vi "MapScriptActorGFV.vi"(8 "error in (no error)":errorcluster, 10 "MapScriptEnum":T1, 11 "Data in":variant) -> (0 "error out":errorcluster, 3 "Data Out":variant)   [LabVIEW 2017]
doc: "Use this template to build a VI to use as a subVI."
uses:
  MapScriptGFVEnum.ctl
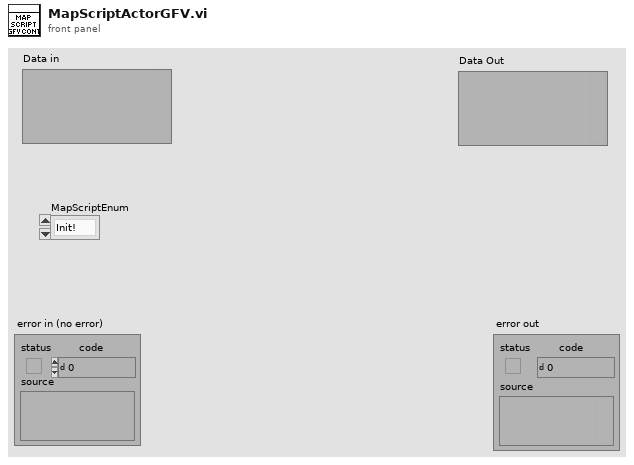
[diagram p1: front panel]
types:
  T1 = typedef "MapScriptGFVEnum.ctl" = enum16{"Init!", "Stop!", "Start!", "GetMapScriptActorViRef"}
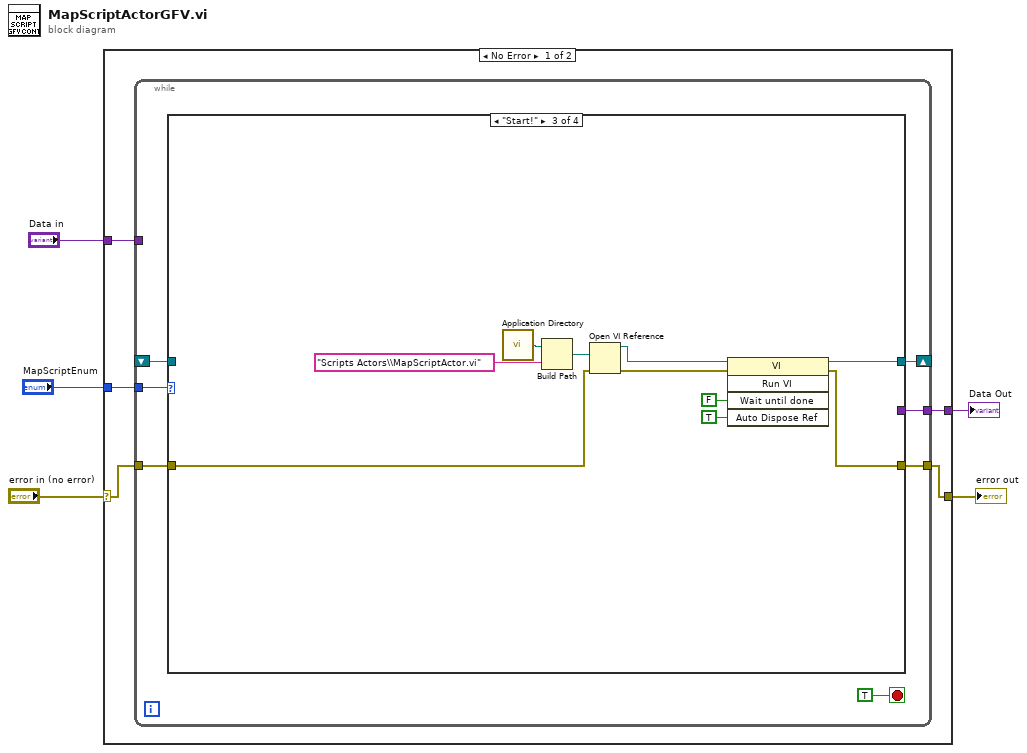
[diagram p0: block diagram]
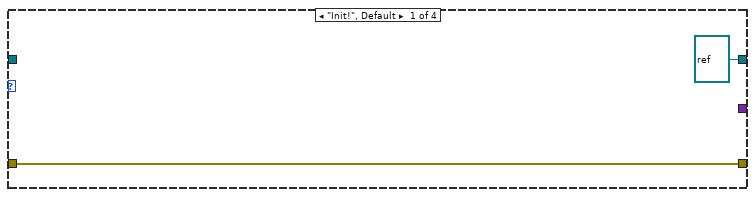
[diagram p2: hidden frame]
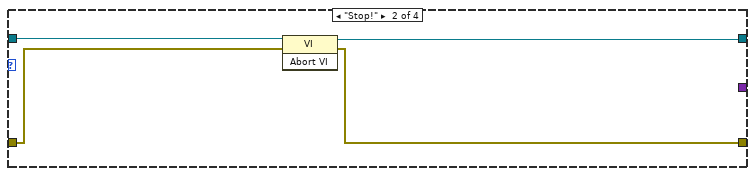
[diagram p3: hidden frame]
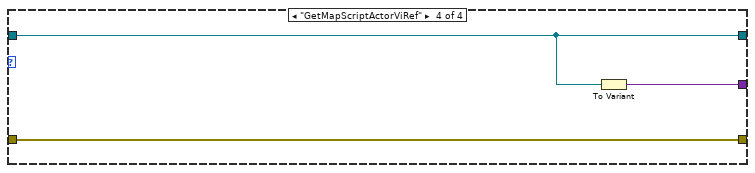
[diagram p4: hidden frame]
diagram:
  n1 = case shown="No Error" "error in (no error)" {
    selector: "error in (no error)" -> [w9 w37]
    tunnel: [w8 w37] -> w4
    tunnel: "MapScriptEnum" -> [w10 _]
    tunnel: "Data in" -> [w7 _]
    tunnel: [w6 _] -> w1
    frame No Error {
      n2 = while {
        tunnel: w10 -> [w16]
        tunnel: w9 -> [w15]
        tunnel: [w14] -> w8
        shift-right: [w13] -> _
        shift-left: _ -> [w12]
        tunnel: w7 -> [_]
        tunnel: [w11] -> w6
        stop <- TRUE stop-if-true
        n3 = case shown="\"Start!\"" w16 {
          tunnel: w15 -> [w18 w23 w26 w34]
          tunnel: [w18 w22 w25 w34] -> w14
          tunnel: [refnum<vi> refnum ("vi reference") w20 w24 w36] -> w13
          tunnel: w12 -> [_ w21 _ w36]
          tunnel: [_ _ _ w35] -> w11
          frame "Init!", Default {
          }
          frame "Stop!" {
            n4 = invoke class="VI" method="Abort VI"(reference=w21, error in=w23) -> (reference out=w20:refnum<vi>, error out=w22:errorcluster)  [unwired: 1 in, 1 out]
          }
          frame "Start!" {
            n5 = call <vilib>:"Application Directory.vi"() -> ("Application Directory"=w31:path)
            n6 = Build Path(base path=w31, name or relative path="Scripts Actors\\MapScriptActor.vi") -> (appended path=w29:path)
            n7 = Open VI Reference(vi path=w29, error in (no error)=w26) -> (vi reference=w27:refnum<vi>, error out=w28:errorcluster)  [unwired: 4 in]
            n8 = invoke class="VI" method="Run VI"(reference=w27, error in=w28, "Wait until done"=FALSE ("Wait Until Done"), "Auto Dispose Ref"=TRUE ("Auto Dispose Reference")) -> (reference out=w24:refnum<vi>, error out=w25:errorcluster)  [unwired: 1 in, 3 out]
          }
          frame "GetMapScriptActorViRef" {
            n9 = To Variant(anything=w36) -> (Variant=w35:variant)
          }
        }
      }
    }
    frame Error {
    }
  }
  "error out" <- w4
  "Data Out" <- w1
